vi "test-ltv-unicycle-controller-Test1.vi"() -> (3 "All tests passed":bool)   [LabVIEW 2019]
uses:
  <vilib>/Rock Robotics/WPI/ThirdParty/JAS_Junk/TrajLib/TRAJECTORY.ctl
  <vilib>/Rock Robotics/WPI/ThirdParty/JAS_Junk/TrajLib/TRAJ_STATE.ctl
  <vilib>/Rock Robotics/WPI/ThirdParty/JAS_Junk/TrajLib/POSE2D.ctl
  <vilib>/Rock Robotics/WPI/ThirdParty/JAS_Junk/TrajLib/TRANSLATION2D.ctl
  <vilib>/Rock Robotics/WPI/ThirdParty/JAS_Junk/TrajLib/ROTATION2D.ctl
  <vilib>/Rock Robotics/WPI/ThirdParty/JAS_Junk/TrajLib/CHASSIS_SPEEDS.ctl
  <vilib>/Rock Robotics/WPI/ThirdParty/JAS_Junk/TrajLib/LTV_UNICYCLE_CONTROLLER.ctl
  <vilib>/Analysis/Matrix/Datatypes/RealMatrix.ctl
  <vilib>/Rock Robotics/WPI/ThirdParty/JAS_Junk/TrajLib/FUNCTION_GENERATOR_MATRIX.ctl
  <vilib>/Rock Robotics/WPI/ThirdParty/JAS_Junk/TrajLib/TRAJECTORY_SPLINE_TYPE_ENUM.ctl
  <vilib>/numeric/Random Number (Range) DBL.vi
  <vilib>/Rock Robotics/WPI/ThirdParty/JAS_Junk/TrajLib/Conv_Inches_Meters.vi
  <vilib>/Rock Robotics/WPI/ThirdParty/JAS_Junk/TrajLib/Rotation2d_CreateAngle.vi
  <vilib>/Rock Robotics/WPI/ThirdParty/JAS_Junk/TrajLib/Translation2d_Create.vi
  <vilib>/Rock Robotics/WPI/ThirdParty/JAS_Junk/TrajLib/MatBuilder_Create.vi
  <vilib>/Rock Robotics/WPI/ThirdParty/JAS_Junk/TrajLib/SlewRateLimiter_New.vi
  <vilib>/Rock Robotics/WPI/ThirdParty/JAS_Junk/TrajLib/SlewRateLimiter_Reset.vi
  <vilib>/Rock Robotics/WPI/ThirdParty/JAS_Junk/TrajLib/SlewRateLimiter_Calculate.vi
  <vilib>/Rock Robotics/WPI/ThirdParty/JAS_Junk/TrajLib/SlewRateLimiter_SetRate.vi
  <vilib>/Rock Robotics/WPI/ThirdParty/JAS_Junk/TrajLib/Util_GetTime.vi
  <vilib>/Rock Robotics/WPI/ThirdParty/JAS_Junk/TrajLib/Trajectory_Library.lvlib
  <vilib>/Analysis/Matrix/NI_Matrix.lvlib
panel:
  in  "Use Rate Limit":bool=TRUE
  in  "Use Noise":bool
  out "Any Calc Error":bool
  out "At Reference":bool
  out "Waveform Graph":dbl[][](graph)
  out "Ctrl":T1={"m_A"=[], "m_B"=[], "m_Q"=[], "m_R"=[], "States"=0, "Inputs"=0, "PoseError"={"TRANSLATION"={"X"=0.0, "Y"=0.0}, "ROTATION"={"VALUE"=0.0, "COS"=1.0, "SIN"=0.0}}, "PoseTolerance"={"TRANSLATION"={"X"=0.0, "Y"=0.0}, "ROTATION"={"VALUE"=0.0, "COS"=1.0, "SIN"=0.0}}, "Dt"=0.02, "Enabled"=FALSE, "savedLQR_K"={"Table Xs"=[], "Table Ys"=[], "MinX"=0.0, "MaxX"=0.0, "ItemCount"=0, "Rows"=0, "Columns"=0}} {"PoseTolerance"."ROTATION"."SIN" format="%13.4f"; "PoseTolerance"."ROTATION"."COS" format="%13.4f"; "PoseTolerance"."ROTATION"."VALUE" format="%13.4f"; "PoseTolerance"."TRANSLATION"."Y" format="%14.3f"; "PoseTolerance"."TRANSLATION"."X" format="%14.3f"; "PoseError"."ROTATION"."SIN" format="%13.4f"; "PoseError"."ROTATION"."COS" format="%13.4f"; "PoseError"."ROTATION"."VALUE" format="%13.4f"; "PoseError"."TRANSLATION"."Y" format="%14.3f"; "PoseError"."TRANSLATION"."X" format="%14.3f"}
  out "ChassisSpeeds":T7 {"vOmega" format="%10.3f"; "vY" format="%10.3f"; "vX" format="%10.3f"}
  out "XY Graph":cluster{dbl[], dbl[]}[](graph)
  out "X":bool
  out "Y":bool
  out "Rot":bool
  out "TotalTime_Sec":dbl
  out "OutputTRAJ_STATE":T8={"TimeSeconds"=0.0, "Velocity"=0.0, "Acceleration"=0.0, "POSE"={"TRANSLATION"={"X"=0.0, "Y"=0.0}, "ROTATION"={"VALUE"=0.0, "COS"=1.0, "SIN"=0.0}}, "Curvature"=0.0} {"POSE"."ROTATION"."SIN" format="%13.4f"; "POSE"."ROTATION"."COS" format="%13.4f"; "POSE"."ROTATION"."VALUE" format="%13.4f"; "POSE"."TRANSLATION"."Y" format="%14.3f"; "POSE"."TRANSLATION"."X" format="%14.3f"}
  out "UpdatedPose":T3 {"ROTATION"."SIN" format="%13.4f"; "ROTATION"."COS" format="%13.4f"; "ROTATION"."VALUE" format="%13.4f"; "TRANSLATION"."Y" format="%14.3f"; "TRANSLATION"."X" format="%14.3f"}
  out "TrajStatePose":T3={"TRANSLATION"={"X"=0.0, "Y"=0.0}, "ROTATION"={"VALUE"=0.0, "COS"=1.0, "SIN"=0.0}} {"ROTATION"."SIN" format="%13.4f"; "ROTATION"."COS" format="%13.4f"; "ROTATION"."VALUE" format="%13.4f"; "TRANSLATION"."Y" format="%14.3f"; "TRANSLATION"."X" format="%14.3f"}
  out "Calc Error":bool
  out "Create\nError":bool
  out "TRAJECTORY":T9 {"States"."POSE"."ROTATION"."SIN" format="%13.4f"; "States"."POSE"."ROTATION"."COS" format="%13.4f"; "States"."POSE"."ROTATION"."VALUE" format="%13.4f"; "States"."POSE"."TRANSLATION"."Y" format="%14.3f"; "States"."POSE"."TRANSLATION"."X" format="%14.3f"; "TotalTImeSecs" format="%20.3f"}
  # "<States,States>"
  # "<States,Inputs>"
  # "<States, States>"
  # "<Inputs, Inputs>"
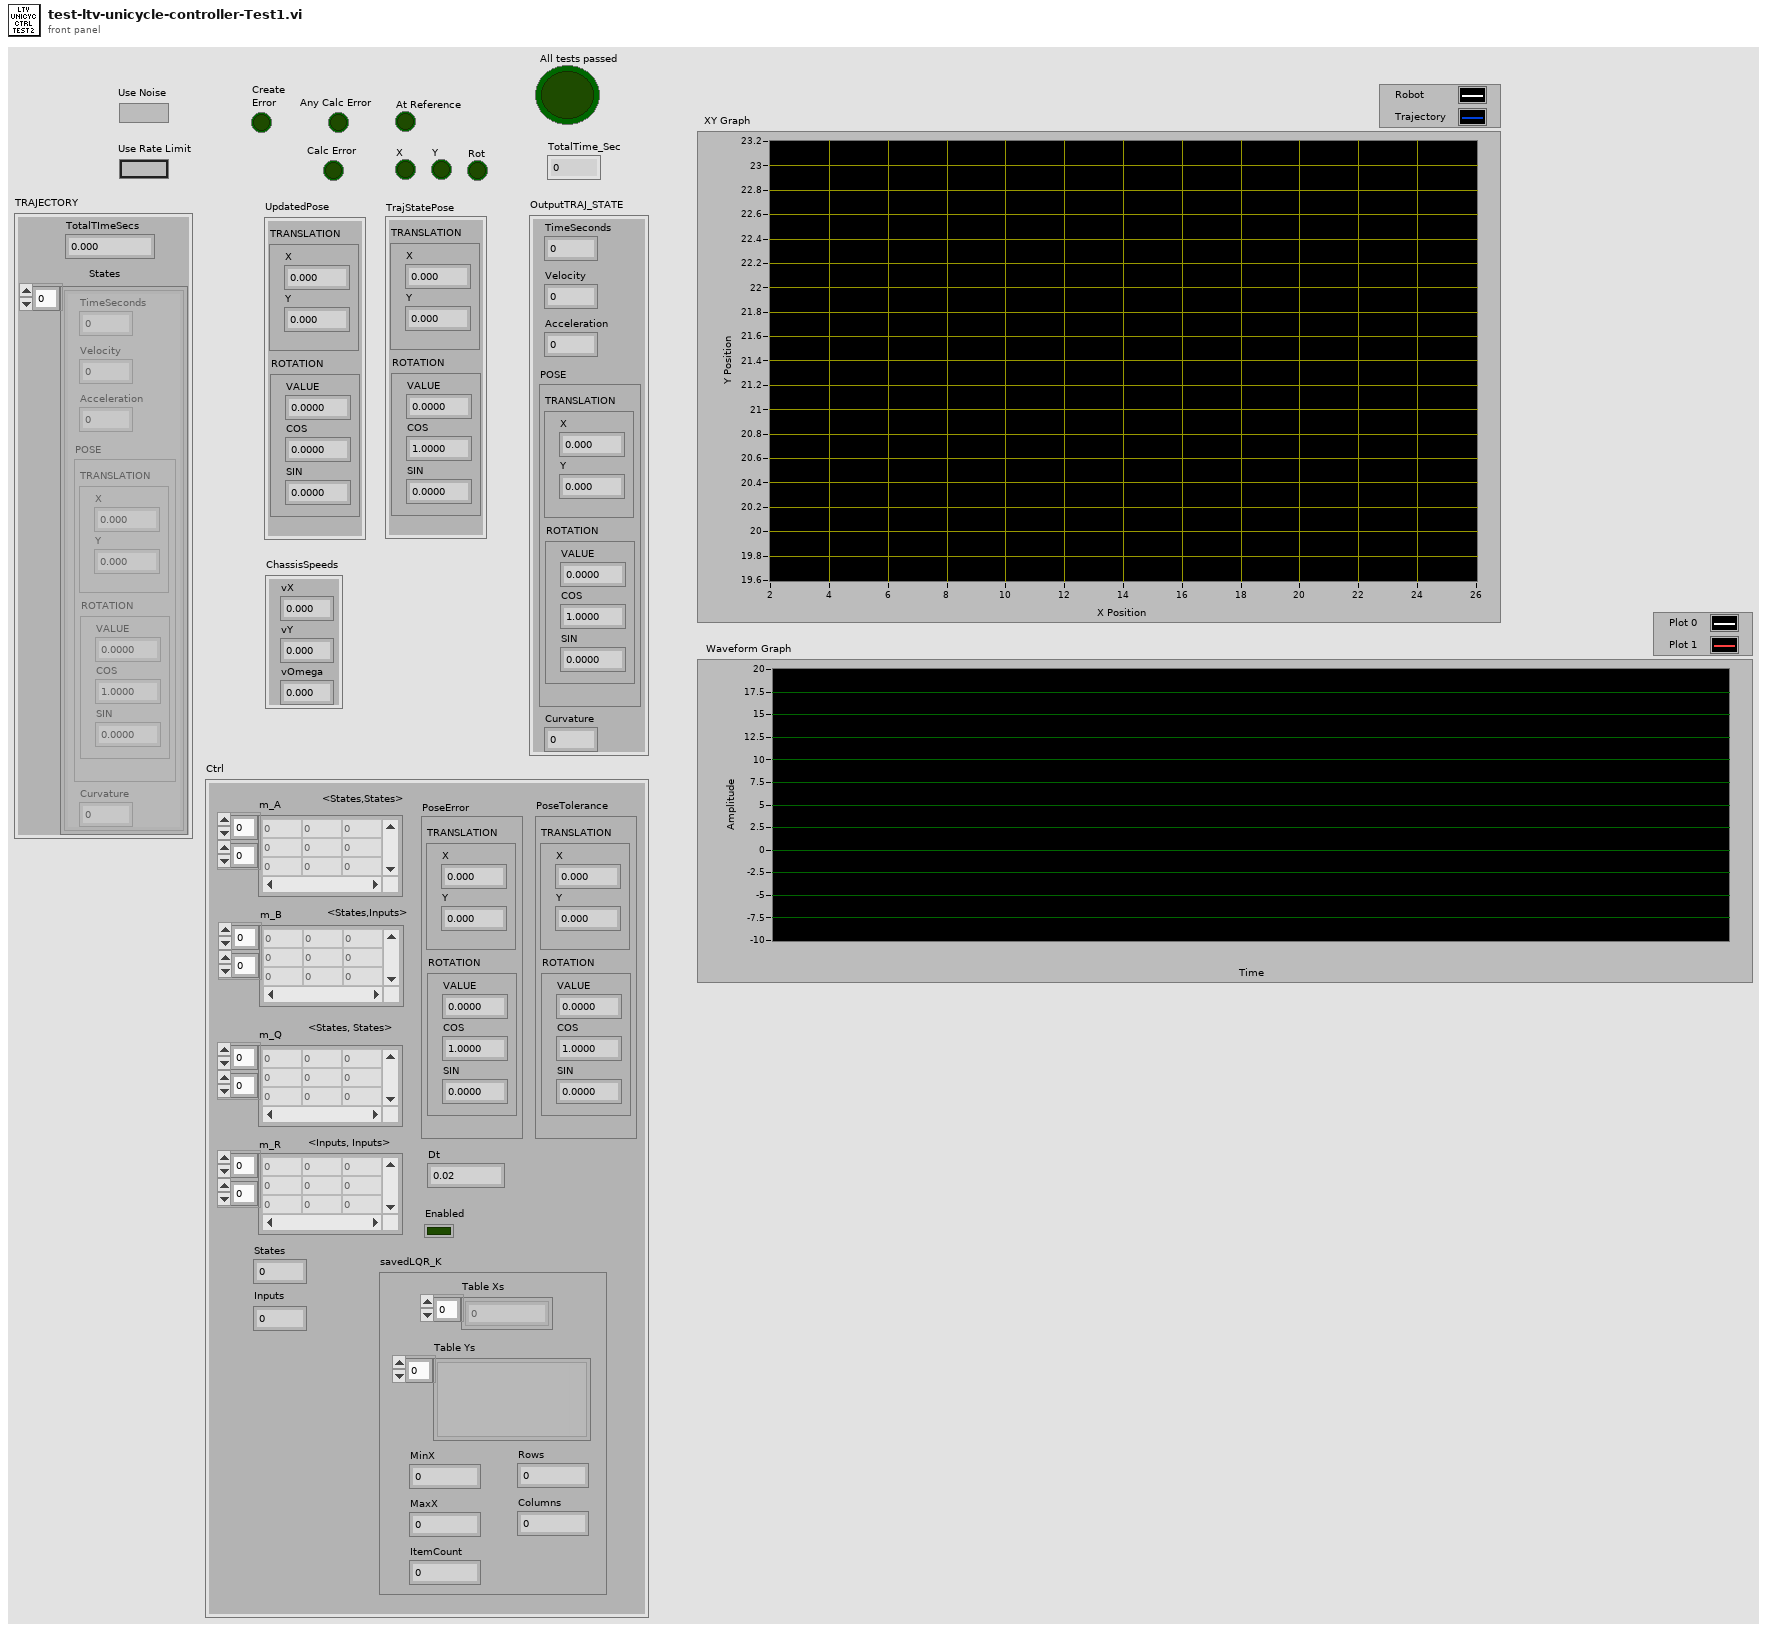
[diagram p1: front panel]
types:
  T1 = typedef "Trajectory_Library.lvlib/LTV_UNICYCLE_CONTROLLER.ctl" = cluster{"m_A":T2, "m_B":T2, "m_Q":T2, "m_R":T2, "States":i32, "Inputs":i32, "PoseError":T3, "PoseTolerance":T3, "Dt":dbl, "Enabled":bool, "savedLQR_K":T6}
  T2 = typedef "NI_Matrix.lvlib/RealMatrix.ctl" = dbl[][]
  T3 = typedef "Trajectory_Library.lvlib/POSE2D.ctl" = cluster{"TRANSLATION":T4, "ROTATION":T5}
  T4 = typedef "Trajectory_Library.lvlib/TRANSLATION2D.ctl" = cluster{"X":dbl, "Y":dbl}
  T5 = typedef "Trajectory_Library.lvlib/ROTATION2D.ctl" = cluster{"VALUE":dbl, "COS":dbl, "SIN":dbl}
  T6 = typedef "Trajectory_Library.lvlib/FUNCTION_GENERATOR_MATRIX.ctl" = cluster{"Table Xs":dbl[], "Table Ys":variant[], "MinX":dbl, "MaxX":dbl, "ItemCount":i32, "Rows":i32, "Columns":i32}
  T7 = typedef "Trajectory_Library.lvlib/CHASSIS_SPEEDS.ctl" = cluster{"vX":dbl, "vY":dbl, "vOmega":dbl}
  T8 = typedef "Trajectory_Library.lvlib/TRAJ_STATE.ctl" = cluster{"TimeSeconds":dbl, "Velocity":dbl, "Acceleration":dbl, "POSE":T3, "Curvature":dbl}
  T9 = typedef "Trajectory_Library.lvlib/TRAJECTORY.ctl" = cluster{"TotalTImeSecs":dbl, "States":T8[]}
  T10 = typedef "Trajectory_Library.lvlib/TRAJECTORY_SPLINE_TYPE_ENUM.ctl" = enum16{"Cubic", "Cubic With Weights", "Quintic", "Quintic With Weights"}
  T11 = typedef "Trajectory_Library.lvlib/WEIGHTED_WAYPOINT.ctl" = cluster{"TRANSLATION":T4, "ROTATION":T5, "SCALAR":dbl}
  T12 = typedef "Trajectory_Library.lvlib/TRAJ_CONFIG.ctl" = cluster{"MaxVelocity":dbl, "Max Acceleration":dbl, "StartVelocity":dbl, "End Velocity":dbl, "Reversed":bool, "DiffDrKineConstntDefined":bool, "CentAcellConstntDefined":bool, "DiffDrVoltConstntDefined":bool, "DIFF_DRIVE_KINE_CONSTRAINT":T13, "CENTRIPETAL_ACCEL_CONSTRAINT":T15, "SwerveDrKineConstntDefined":bool, "SWERVE_DRIVE_KINE_CONSTRAINT":T16, "DIFF_DRIVE_VOLTAGE_CONSTRAINT":T18, "MECANUM_DRIVE_KINE_CONSTRAINT":T20, "MecanumDrKineConstntDefined":bool}
  T13 = typedef "Trajectory_Library.lvlib/TRAJ_CONSTRAINT_DIIF_DRIVE_KINEMATICS.ctl" = cluster{"Max Speed (M/S)":dbl, "DIFF_DRIVE_KINEMATICS":T14, "Max Accel (M/S2)":dbl}
  T14 = typedef "Trajectory_Library.lvlib/DIFF_DRIVE_KINEMATICS.ctl" = cluster{"TrackWidth_Meters":dbl}
  T15 = typedef "Trajectory_Library.lvlib/TRAJ_CONSTRAINT_CENTRIPETAL_ACCEL.ctl" = cluster{"Max Cent Accel":dbl}
  T16 = typedef "Trajectory_Library.lvlib/TRAJ_CONSTRAINT_SWERVE_DRIVE_KINEMATICS.ctl" = cluster{"Max Speed (M/S)":dbl, "SwerveKinematics":T17}
  T17 = typedef "Trajectory_Library.lvlib/SWERVE_DRIVE_KINEMATICS.ctl" = cluster{"NumModules":i32, "InverseKinematics":T2, "ForwardKinematics":T2, "Modules":T4[], "PrevCoR":T4}
  T18 = typedef "Trajectory_Library.lvlib/TRAJ_CONSTRAINT_DIIF_DRIVE_VOLTAGE.ctl" = cluster{"Max Voltage":dbl, "DIFF_DRIVE_KINEMATICS":T14, "SIMPLE_MOTOR_FF":T19}
  T19 = typedef "Trajectory_Library.lvlib/SIMPLE_MOTOR_FF.ctl" = cluster{"Ks":dbl, "Kv":dbl, "Ka":dbl}
  T20 = typedef "Trajectory_Library.lvlib/TRAJ_CONSTRAINT_MECA_DRIVE_KINEMATICS.ctl" = cluster{"Max Speed (M/S)":dbl, "MECA_DRIVE_KINEMATICS":T21}
  T21 = typedef "Trajectory_Library.lvlib/MECA_DRIVE_KINEMATICS.ctl" = cluster{"FrontLeft":T4, "FrontRight":T4, "RearLeft":T4, "RearRight":T4, "InverseKinematics":T2, "ForwardKinematics":T2, "PrevCoR":T4}
  T22 = typedef "Trajectory_Library.lvlib/TWIST2D.ctl" = cluster{"dX":dbl, "dY":dbl, "dTHETA":dbl}
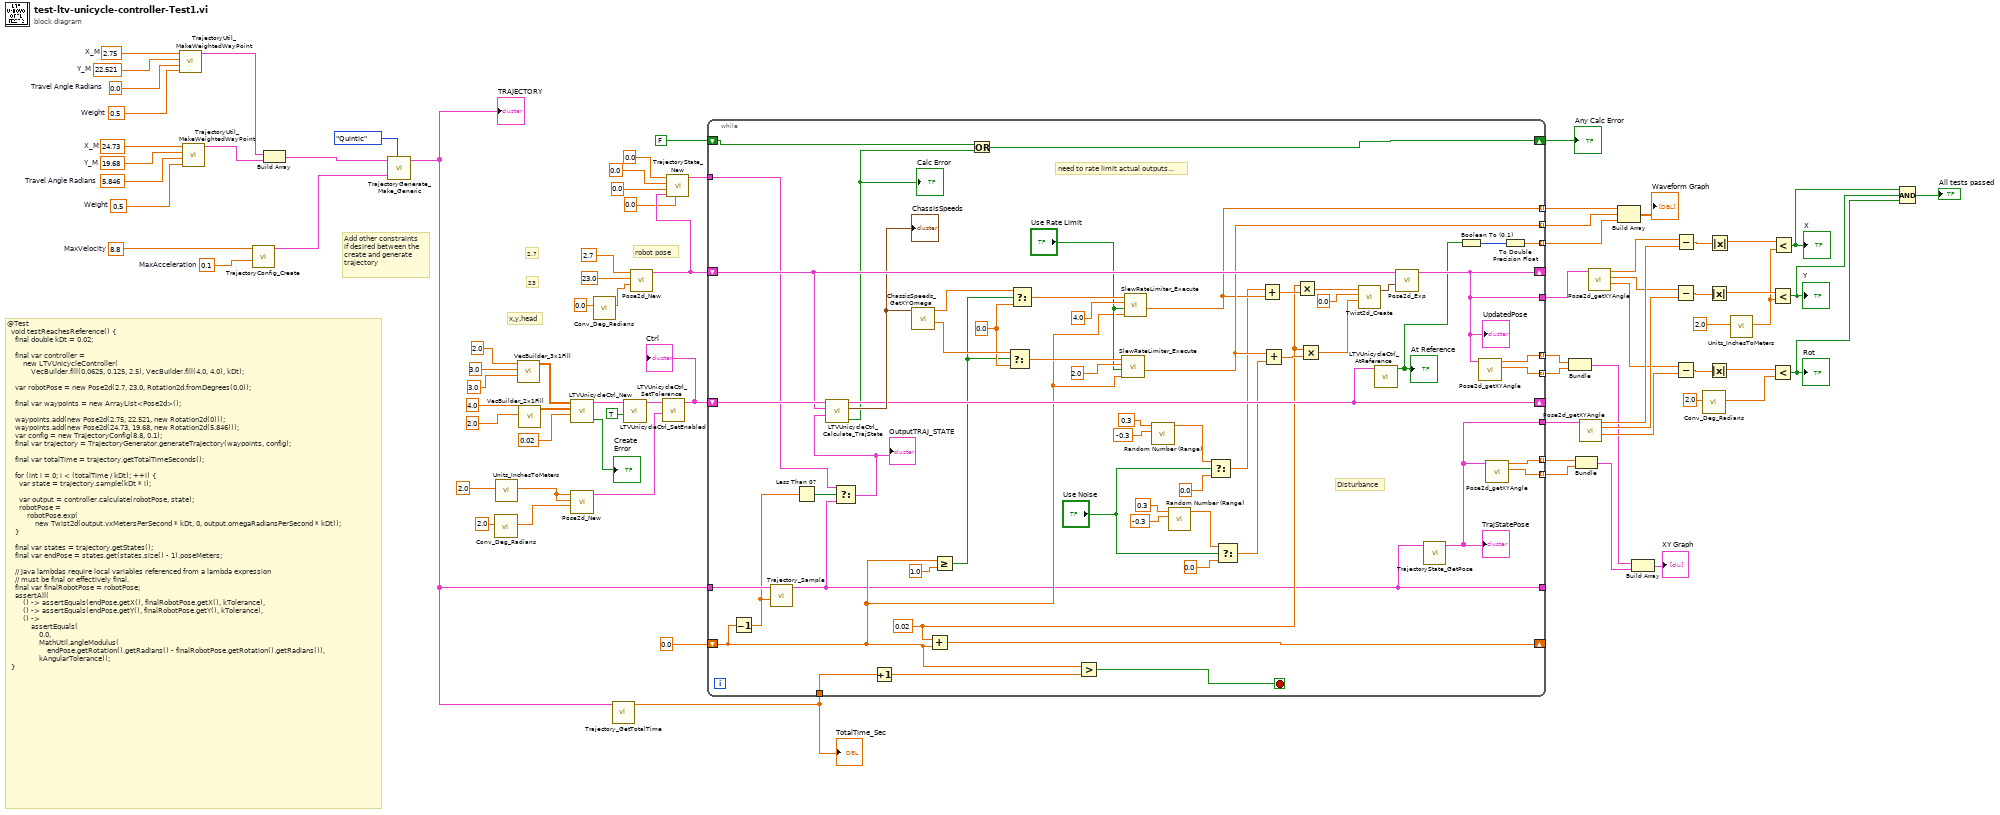
[diagram p0: block diagram]
diagram:
  w68 = 24.73  # X_M
  w67 = 19.68  # Y_M
  w55 = 5.846  # Travel Angle Radians
  w66 = 0.5  # Weight
  w65 = 2.75  # X_M
  w64 = 22.521  # Y_M
  w56 = 0.0  # Travel Angle Radians
  w63 = 0.5  # Weight
  w62 = 8.8  # MaxVelocity
  w61 = 0.1  # MaxAcceleration
  # "23"
  # "2.7"
  # "x,y,head"
  # "@Test\n  void testReachesReference() {\n    final double kDt = 0.02;\n\n    final var controller =\n        new LTVUnicycleController(\n            VecBuilder.fill(0.0625, 0.125, 2.5), VecBuilder.fill(4.0, 4.0), kDt);\n\n    var robotPose = new Pose2d(2.7, 23.0, Rotation2d.fromDegrees(0.0));\n\n    final var waypoints = new ArrayList<Pose2d>();\n\n    waypoints.add(new Pose2d(2.75, 22.521, new Rotation2d(0)));\n    waypoints.add(new Pose2d(24.73, 19.68, new Rotation2d(5.846)));\n    var config = new TrajectoryConfig(8.8, 0.1);\n    final var trajectory = TrajectoryGenerator.generateTrajectory(waypoints, config);\n\n    final var totalTime = trajectory.getTotalTimeSeconds();\n\n    for (int i = 0; i < (totalTime / kDt); ++i) {\n      var state = trajectory.sample(kDt * i);\n\n      var output = controller.calculate(robotPose, state);\n      robotPose =\n          robotPose.exp(\n              new Twist2d(output.vxMetersPerSecond * kDt, 0, output.omegaRadiansPerSecond * kDt));\n    }\n\n    final var states = trajectory.getStates();\n    final var endPose = states.get(states.size() - 1).poseMeters;\n\n    // Java lambdas require local variables referenced from a lambda expression\n    // must be final or effectively final.\n    final var finalRobotPose = robotPose;\n    assertAll(\n        () -> assertEquals(endPose.getX(), finalRobotPose.getX(), kTolerance),\n        () -> assertEquals(endPose.getY(), finalRobotPose.getY(), kTolerance),\n        () ->\n            assertEquals(\n                0.0,\n                MathUtil.angleModulus(\n                    endPose.getRotation().getRadians() - finalRobotPose.getRotation().getRadians()),\n                kAngularTolerance));\n  }"
  # "Add other constraints\nif desired between the\ncreate and generate\ntrajectory"
  # "robot pose"
  n1 = call <vilib>:"TrajectoryUtil_MakeWeightedWayPoint.vi"("Weight"=w63, "Travel Angle Radians"=w56, "Y_M"=w64, "X_M"=w65) -> ("WEIGHTED_WAYPOINT"=w57:T11)  [unwired: 7 in]
  n2 = call <vilib>:"TrajectoryUtil_MakeWeightedWayPoint.vi"("Weight"=w66, "Travel Angle Radians"=w55, "Y_M"=w67, "X_M"=w68) -> ("WEIGHTED_WAYPOINT"=w69:T11)  [unwired: 7 in]
  n3 = call <vilib>:"TrajectoryConfig_Create.vi"("MaxAcceleration"=w61, "MaxVelocity"=w62) -> ("TRAJECTORY_CONFIG"=w60:T12)  [unwired: 9 in]
  n4 = Build Array(w57, w69) -> (w58:T11[])
  n5 = call <vilib>:"TrajectoryGenerate_Make_Generic.vi"("Spline Type"=TRAJECTORY_SPLINE_TYPE_ENUM."Quintic", "traj_config"=w60, "WeightedWayPoints"=w58) -> ("TRAJECTORY"=w52:T9)  [unwired: 7 in, 1 out]
  "TRAJECTORY" <- w52
  n6 = call <vilib>:"Conv_Deg_Radians.vi"("Degress"=2.0) -> ("Radians"=w19:dbl)  [unwired: 10 in]
  n7 = call <vilib>:"Units_InchesToMeters.vi"("Inches"=2.0 ("x")) -> ("Meters"=w8:dbl)  [unwired: 10 in]
  n8 = call <vilib>:"VecBuilder_3x1Fill.vi"("R2"=3.0, "R1"=3.0, "R0"=2.0) -> ("output matrix"=w80:T2)  [unwired: 8 in]
  n9 = call <vilib>:"VecBuilder_2x1Fill.vi"("R1"=2.0, "R0"=4.0) -> ("output matrix"=w79:T2)  [unwired: 9 in]
  n10 = call <vilib>:"LTVUnicycleCtrl_New.vi"("dT"=0.02, "RELMS"=w79, "QELMS"=w80) -> ("Error"=→"Create\nError":bool, "LTV_UNICYCLE_CONTROLLER"=w27:T1)  [unwired: 7 in]
  n11 = call <vilib>:"Pose2d_New.vi"("Heading"=w19, "Y"=w8, "X"=w8) -> ("out POSe"=w18:T3)  [unwired: 8 in]
  n12 = call <vilib>:"Conv_Deg_Radians.vi"("Degress"=0.0) -> ("Radians"=w73:dbl)  [unwired: 10 in]
  n13 = call <vilib>:"Trajectory_GetTotalTime.vi"("TRAJECTORY"=w52) -> ("TotalTime_Sec"=w53:dbl)  [unwired: 10 in]
  "TotalTime_Sec" <- w53
  n14 = call <vilib>:"LTVUnicycleCtrl_SetEnabled.vi"("Enabled"=TRUE, "in LTV_UNICYCLE_CONTROLLER"=w27) -> ("out LTV_UNICYCLE_CONTROLLER"=w21:T1)  [unwired: 9 in]
  n15 = call <vilib>:"Pose2d_New.vi"("Heading"=w73, "Y"=23.0, "X"=2.7) -> ("out POSe"=w6:T3)  [unwired: 8 in]
  n16 = call <vilib>:"LTVUnicycleCtrl_SetTolerance.vi"("Tolerance"=w18, "in LTV_UNICYCLE_CONTROLLER"=w21) -> ("out LTV_UNICYCLE_CONTROLLER"=w20:T1)  [unwired: 9 in]
  "Ctrl" <- w20
  n17 = call <vilib>:"TrajectoryState_New.vi"("Curvature"=0.0, "POSE"=w6, "Accel"=0.0, "Velocity"=0.0, "Time"=0.0) -> ("TRAJ_STATE"=w1:T8)  [unwired: 6 in]
  n18 = while {
    shift-right: [w137] -> _
    shift-left: 0.0 -> [w88]
    tunnel: w53 -> [w90]
    tunnel: w52 -> [w136]
    shift-right: [w124] -> _
    shift-left: w6 -> [w134]
    shift-right: [w120] -> _
    shift-left: w20 -> [w135]
    tunnel: [w86] -> _
    tunnel: [w123] -> w50
    tunnel: [w128] -> w35 mode=indexing
    tunnel: [w127] -> w34 mode=indexing
    tunnel: [w126] -> w33 mode=indexing
    tunnel: [w125] -> w32 mode=indexing
    tunnel: [w124] -> w28
    tunnel: [w114] -> w25 mode=indexing
    tunnel: [w116] -> w23 mode=indexing
    tunnel: [w117] -> w17 mode=indexing
    shift-right: [w106] -> w11
    shift-left: FALSE -> [w108]
    tunnel: w1 -> [w82]
    stop <- w138 stop-if-true
    w93 = 0.0 ("f")
    w98 = 0.02 ("x")
    # "Disturbance"
    # "need to rate limit actual outputs..."
    n19 = Decrement(x=w88) -> (x-1=w84:dbl)
    n20 = call <vilib>:"Trajectory_Sample.vi"("Time"=w84, "InputTRAJECTORY"=w136) -> ("OutputTRAJ_STATE"=w86:T8)  [unwired: 9 in]
    n21 = Less Than 0?(x=w84) -> (x < 0?=w85:bool)
    n22 = Select(t=w82, s=w85, f=w86) -> (s? t:f=w83:T8)
    "OutputTRAJ_STATE" <- w83
    n23 = call <vilib>:"LTVUnicycleCtrl_Calculate_TrajState.vi"("TRAJ_STATE"=w83, "CurrentPose"=w134, "in LTV_UNICYCLE_CONTROLLER"=w135) -> ("Error"=w107:bool, "ChassisSpeeds"=w132:T7, "out LTV_UNICYCLE_CONTROLLER"=w120:T1)  [unwired: 6 in]
    "Calc Error" <- w107
    "ChassisSpeeds" <- w132
    n24 = Increment(x=w90) -> (x+1=w89:dbl)
    n25 = call <vilib>:"ChassisSpeeds_GetXYOmega.vi"("CHASSIS"=w132) -> ("vAngular"=w94:dbl, "vX"=w95:dbl)  [unwired: 8 in, 1 out]
    n26 = Add(x=w98, y=w88) -> (x+y=w137:dbl)
    n27 = Greater Or Equal?(x=w88, y=1.0) -> (x >= y?=w92:bool)
    n28 = Or(x=w108, y=w107) -> (x .or. y?=w106:bool)
    n29 = Select(t=w94, s=w92, f=w93) -> (s? t:f=w97:dbl)
    n30 = Select(t=w95, s=w92, f=w93) -> (s? t:f=w96:dbl)
    n31 = Greater?(x=w88, y=w89) -> (0:w138:bool)
    n32 = call <vilib>:"SlewRateLimiter_Execute.vi"("Time"=w88, "Enable"="Use Rate Limit", "Rate"=2.0, "Input"=w97) -> ("Output"=w116:dbl)  [unwired: 6 in, 1 out]
    n33 = call <vilib>:"SlewRateLimiter_Execute.vi"("Time"=w88, "Enable"="Use Rate Limit", "Rate"=4.0, "Input"=w96) -> ("Output"=w114:dbl)  [unwired: 6 in, 1 out]
    n34 = call-poly <vilib>:"Random Number (Range).vi"("lower bound (0)"=-0.3, "upper bound (100)"=0.3) -> ("number"=w103:dbl)  [unwired: 9 in]
    n35 = call-poly <vilib>:"Random Number (Range).vi"("lower bound (0)"=-0.3, "upper bound (100)"=0.3) -> ("number"=w100:dbl)  [unwired: 9 in]
    n36 = Select(t=w103, s="Use Noise", f=0.0) -> (s? t:f=w105:dbl)
    n37 = Select(t=w100, s="Use Noise", f=0.0) -> (s? t:f=w101:dbl)
    n38 = Add(x=w105, y=w114) -> (x+y=w113:dbl)
    n39 = Add(x=w116, y=w101) -> (x+y=w115:dbl)
    n40 = Multiply(x=w98, y=w113) -> (x*y=w131:dbl)
    n41 = Multiply(x=w98, y=w115) -> (x*y=w129:dbl)
    n42 = call <vilib>:"Twist2d_Create.vi"("dTHETA"=w129, "dY"=0.0, "dX"=w131) -> ("TWIST"=w133:T22)  [unwired: 8 in]
    n43 = call <vilib>:"LTVUnicycleCtrl_AtReference.vi"("LTV_UNICYCLE_CONTROLLER"=w120) -> ("At Reference"=w119:bool)  [unwired: 10 in]
    "At Reference" <- w119
    n44 = call <vilib>:"Pose2d_Exp.vi"("TWIST"=w133, "POSE"=w134) -> ("UpdatedPose"=w124:T3)  [unwired: 9 in]
    "UpdatedPose" <- w124
    n45 = call <vilib>:"TrajectoryState_GetPose.vi"("TRAJ_STATE"=w86) -> ("TrajStatePose"=w123:T3)  [unwired: 10 in]
    "TrajStatePose" <- w123
    n46 = Boolean To (0,1)(Boolean=w119) -> (0, 1=w118:i16)
    n47 = call <vilib>:"Pose2d_getXYAngle.vi"("in POSE"=w124) -> ("Y"=w127:dbl, "X"=w128:dbl)  [unwired: 8 in, 1 out]
    n48 = call <vilib>:"Pose2d_getXYAngle.vi"("in POSE"=w123) -> ("Y"=w125:dbl, "X"=w126:dbl)  [unwired: 8 in, 1 out]
    n49 = To Double Precision Float(number=w118) -> (double precision float=w117:dbl)
  }
  "Any Calc Error" <- w11
  n50 = Bundle(w35, w34) -> (w31:cluster{dbl[], dbl[]})  [unwired: 1 in]
  n51 = Bundle(w33, w32) -> (w30:cluster{dbl[], dbl[]})  [unwired: 1 in]
  n52 = call <vilib>:"Pose2d_getXYAngle.vi"("in POSE"=w50) -> ("Angle"=w38:dbl, "Y"=w40:dbl, "X"=w46:dbl)  [unwired: 8 in]
  n53 = call <vilib>:"Pose2d_getXYAngle.vi"("in POSE"=w28) -> ("Angle"=w39:dbl, "Y"=w41:dbl, "X"=w47:dbl)  [unwired: 8 in]
  n54 = Build Array(w25, w23, w17) -> (→"Waveform Graph":dbl[][])
  n55 = Build Array(w31, w30) -> (→"XY Graph":cluster{dbl[], dbl[]}[])
  n56 = Subtract(x=w41, y=w40) -> (x-y=w44:dbl)
  n57 = Subtract(x=w39, y=w38) -> (x-y=w42:dbl)
  n58 = Subtract(x=w47, y=w46) -> (x-y=w48:dbl)
  n59 = call <vilib>:"Conv_Deg_Radians.vi"("Degress"=2.0) -> ("Radians"=w36:dbl)  [unwired: 10 in]
  n60 = Absolute Value(x=w44) -> (abs(x)=w45:dbl)
  n61 = Absolute Value(x=w42) -> (abs(x)=w43:dbl)
  n62 = Absolute Value(x=w48) -> (abs(x)=w49:dbl)
  n63 = call <vilib>:"Units_InchesToMeters.vi"("Inches"=2.0 ("x")) -> ("Meters"=w10:dbl)  [unwired: 10 in]
  n64 = Less?(x=w45, y=w10) -> (x < y?=w14:bool)
  "Y" <- w14
  n65 = Less?(x=w43, y=w36) -> (x < y?=w13:bool)
  "Rot" <- w13
  n66 = Less?(x=w49, y=w10) -> (x < y?=w15:bool)
  "X" <- w15
  n67 = Compound Arithmetic op=AND(w15, w14, w13) -> (→"All tests passed":bool)
